vi "2024_day02.vi"() -> ()   [LabVIEW 2023]
uses:
  <userlib>/_OpenG.lib/string/string.llb/openg_string.lvlib
panel:
  out "Result - Task 2":i16
  out "Result - Task 1":i16
  in  "Switch":bool caption="Ex. Data  vs.  User Data"
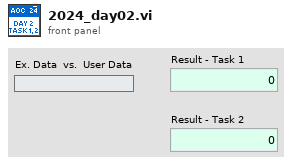
[diagram p1: front panel]
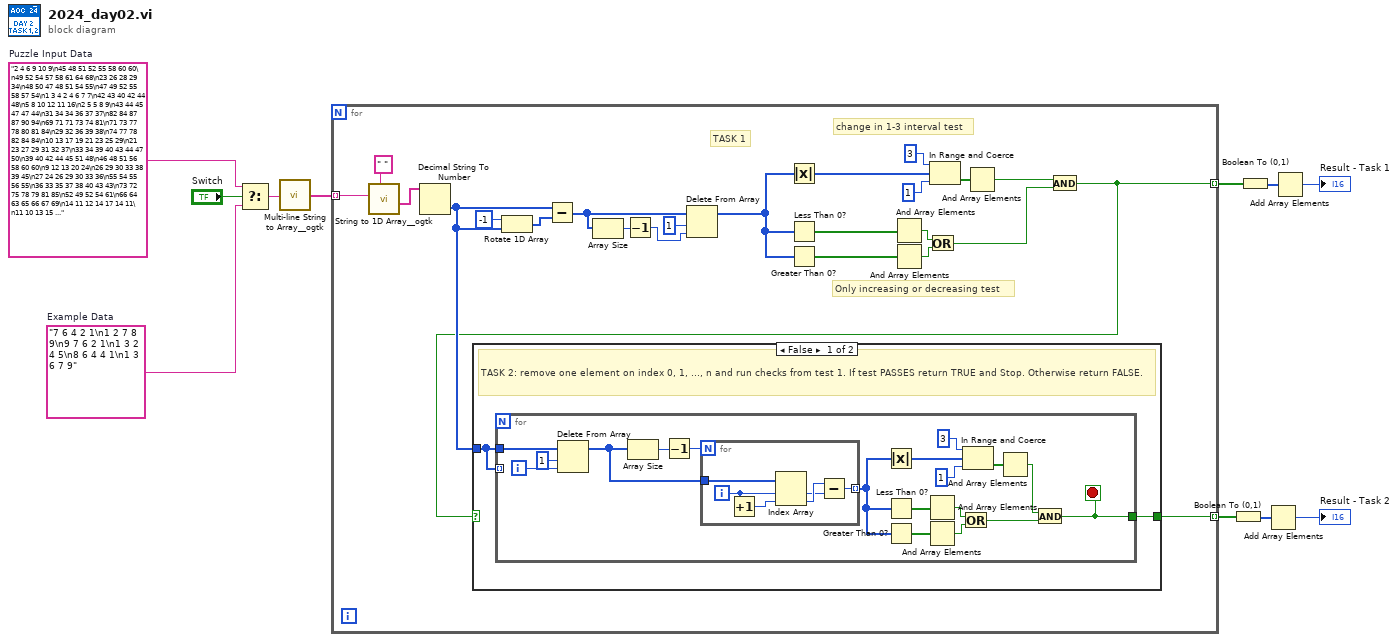
[diagram p0: block diagram]
diagram:
  w9 = "2 4 6 9 10 9\n45 48 51 52 55 58 60 60\n49 52 54 57 58 61 64 68\n23 26 28 29 34\n48 50 47 48 51 54 55\n47 49 52 55 58 57 54\n1 3 4 2 4 6 7 7\n42 43 40 42 44 48\n5 8 10 12 11 16\n2 5 5 8 9\n43 44 45 47 47 44\n31 34 34 36 37 37\n82 84 87 87 90 94\n69 71 71 73 74 81\n71 73 77 78 80 81 84\n29 32 36 39 38\n74 77 78 82 84 84\n10 13 17 19 21 23 25 29\n21 23 27 29 31 32 37\n33 34 39 40 43 44 47 50\n39 40 42 44 45 51 48\n46 48 51 56 58 60 60\n9 12 13 20 24\n26 29 30 33 38 39 45\n27 24 26 29 30 33 36\n55 54 55 56 55\n36 33 35 37 38 40 43 43\n73 72 75 78 79 81 85\n52 49 52 54 61\n66 64 63 65 66 67 69\n14 11 12 14 17 14 11\n11 10 13 15 14 14\n41 38 39 40 38 42\n91 88 86 87 92\n47 44 46 47 48 48 50\n91 89 92 93 93 90\n40 37 37 38 41 41\n60 59 60 63 65 68 68 72\n28 27 28 28 33\n74 71 73 74 76 80 81\n30 28 32 34 32\n51 50 53 54 55 58 62 62\n68 67 70 72 76 80\n17 14 15 19 25\n74 72 75 78 84 87 90 92\n34 32 38 41 42 41\n12 11 12 15 18 24 25 25\n75 74 75 78 79 86 90\n81 78 84 87 88 89 94\n72 72 73 76 78\n22 22 23 24 25 28 26\n47 47 49 50 53 55 55\n19 19 20 23 26 28 32\n23 23 26 27 28 30 32 39\n93 93 94 97 94 96 99\n80 80 83 84 87 84 81\n27 27 30 31 28 31 33 33\n18 18 21 18 22\n51 51 54 51 52 53 60\n24 24 24 27 30\n79 79 79 80 77\n81 81 84 84 86 89 89\n46 46 46 49 52 56\n46 46 46 47 48 54\n40 40 44 47 49 50 53 56\n42 42 45 49 52 54 51\n21 21 24 28 31 31\n66 66 70 71 74 78\n79 79 81 82 83 85 89 94\n18 18 21 26 27\n53 53 58 61 62 59\n57 57 59 61 67 67\n83 83 84 90 94\n4 4 6 11 17\n12 16 17 18 21 24 27 30\n28 32 35 36 38 37\n18 22 25 26 26\n74 78 81 84 86 89 93\n5 9 10 12 13 15 18 23\n57 61 60 63 66\n69 73 74 77 75 76 78 75\n30 34 31 32 32\n77 81 84 86 84 88\n8 12 14 13 15 18 20 26\n61 65 65 66 69\n3 7 10 10 13 15 12\n84 88 90 92 94 94 94\n19 23 26 29 30 30 34\n68 72 75 75 80\n58 62 66 69 71\n9 13 17 18 21 22 19\n7 11 15 16 19 22 22\n23 27 29 33 34 38\n62 66 68 72 78\n54 58 64 67 70 73 74 77\n69 73 78 81 78\n67 71 77 80 83 84 84\n70 74 75 80 84\n40 44 50 51 53 56 61\n65 70 73 75 77\n33 38 40 42 44 43\n43 50 52 53 53\n33 38 41 43 44 48\n72 79 82 85 87 89 92 99\n74 79 81 84 87 84 85\n13 19 21 18 19 16\n89 95 92 94 97 98 98\n35 41 44 47 48 46 50\n35 40 43 41 48\n8 14 16 18 18 19 20\n40 47 49 50 50 51 54 52\n21 26 28 29 29 30 33 33\n40 45 47 48 48 52\n48 53 55 55 61\n54 59 60 64 66 67 68\n35 42 44 46 47 51 49\n40 45 47 51 53 53\n17 22 26 27 31\n75 81 85 87 94\n44 50 57 60 63 65\n48 53 56 63 60\n47 52 54 59 61 61\n27 33 38 41 45\n66 71 72 77 80 83 90\n30 28 27 24 22 21 24\n17 16 15 13 11 8 7 7\n37 36 34 33 31 30 29 25\n93 91 90 87 80\n18 16 15 13 14 11\n77 74 71 70 67 69 70\n49 46 45 44 47 47\n80 79 77 76 77 74 70\n50 49 47 50 49 48 47 42\n86 83 80 80 77\n66 64 61 61 59 57 55 57\n62 60 58 58 55 53 53\n63 60 60 57 53\n59 57 57 56 53 50 48 41\n98 96 92 91 89 88 87\n98 95 91 89 86 88\n78 77 74 72 69 65 65\n15 13 12 10 9 5 1\n62 59 58 54 47\n99 98 97 92 89\n84 83 82 76 75 73 76\n47 44 39 36 35 33 33\n42 39 33 30 29 26 22\n34 32 31 29 27 21 19 13\n55 56 55 54 52\n86 89 88 85 82 83\n72 74 73 70 69 66 66\n70 72 70 68 65 63 60 56\n82 83 82 79 77 76 73 68\n38 41 44 43 40 38\n2 5 4 7 4 5\n79 81 80 83 83\n26 27 24 27 24 23 19\n22 25 26 23 21 18 16 9\n18 21 19 17 17 16\n52 55 53 53 50 49 51\n25 27 26 26 23 21 21\n9 11 8 8 4\n23 26 23 21 21 18 17 12\n54 55 53 51 47 45\n79 82 80 76 75 73 71 72\n69 71 67 64 62 60 60\n26 29 28 24 20\n71 74 70 69 67 64 58\n82 83 76 75 74 73 72\n79 82 80 75 73 75\n7 10 5 3 1 1\n84 87 86 80 78 75 71\n27 28 21 20 17 15 8\n90 90 89 86 84\n35 35 34 32 31 29 26 28\n57 57 55 54 52 49 49\n51 51 50 47 43\n65 65 63 61 59 58 57 52\n44 44 43 40 37 35 38 35\n24 24 22 20 18 21 18 19\n76 76 75 78 78\n39 39 36 39 36 35 31\n39 39 40 38 31\n28 28 25 22 22 19\n12 12 9 8 8 6 4 7\n19 19 16 16 16\n63 63 62 59 59 55\n87 87 87 85 78\n64 64 61 57 55 53 50\n61 61 58 54 56\n17 17 14 10 8 8\n48 48 46 42 41 40 39 35\n29 29 25 22 17\n60 60 57 55 52 47 44\n63 63 62 60 54 53 51 52\n98 98 92 91 91\n46 46 43 41 38 32 28\n37 37 32 29 26 23 21 14\n57 53 52 49 48 46 45\n85 81 79 78 76 78\n24 20 17 16 13 12 9 9\n39 35 34 32 28\n56 52 50 47 46 45 44 38\n13 9 11 9 6\n98 94 92 90 92 90 89 90\n28 24 25 22 20 20\n42 38 35 33 35 33 29\n23 19 17 18 17 14 12 6\n35 31 29 26 25 25 24 23\n23 19 16 14 11 8 8 11\n82 78 78 76 76\n44 40 40 37 33\n45 41 39 38 38 31\n77 73 70 68 64 63 62\n52 48 47 43 40 39 38 40\n74 70 66 63 63\n55 51 47 46 45 44 40\n71 67 64 63 59 58 57 52\n49 45 43 40 39 36 30 28\n44 40 37 35 29 31\n27 23 21 20 19 16 11 11\n55 51 46 45 41\n83 79 77 71 70 68 62\n16 9 7 4 3\n67 62 60 57 58\n30 24 21 19 18 17 14 14\n21 15 13 11 7\n27 22 20 19 16 13 11 5\n15 8 7 8 5\n53 46 43 40 41 38 39\n76 70 69 66 68 68\n39 32 34 32 29 26 25 21\n92 85 83 86 84 81 76\n27 20 18 17 16 16 15\n21 14 11 9 8 8 9\n27 22 21 21 19 19\n58 53 53 51 48 47 43\n66 59 56 56 53 46\n70 64 60 59 56\n48 43 40 39 35 38\n61 54 50 48 46 46\n72 67 63 62 61 60 56\n96 91 87 84 77\n60 55 50 48 47 45\n43 38 35 29 28 25 27\n94 89 88 86 84 78 77 77\n58 51 48 46 43 41 34 30\n35 29 26 20 13\n87 90 91 92 89\n9 10 11 13 15 15\n5 6 7 8 11 14 15 19\n61 64 66 68 69 76\n64 66 67 69 71 74 73 75\n13 14 17 16 18 17\n91 94 97 94 96 96\n87 88 87 88 90 93 97\n47 49 51 48 53\n29 30 33 35 38 40 40 41\n58 61 62 65 68 68 71 69\n4 6 9 9 9\n73 76 77 79 79 81 85\n30 32 34 34 39\n24 27 30 31 35 38 41\n69 72 76 78 77\n29 31 33 37 37\n66 68 70 72 76 80\n82 84 87 91 98\n68 71 74 79 81 84 86\n72 75 77 78 81 86 88 86\n11 14 20 21 21\n44 46 48 49 50 56 57 61\n31 34 35 38 40 41 48 53\n56 53 55 56 58 60\n56 53 56 59 61 62 61\n9 8 10 13 13\n7 4 5 8 9 11 15\n29 27 29 32 38\n10 8 10 11 10 13\n77 74 77 76 73\n80 79 81 83 82 84 84\n68 65 67 64 68\n45 44 41 44 46 47 50 57\n15 14 16 17 17 19 22 23\n28 26 27 27 25\n67 64 64 67 70 70\n10 7 10 12 12 13 17\n56 54 54 55 62\n23 20 22 26 27 30\n29 28 31 35 33\n21 19 23 25 25\n37 35 39 42 43 47\n60 57 61 64 69\n49 47 54 57 58 59 60\n76 74 79 81 78\n60 57 58 64 67 67\n59 57 64 65 69\n80 77 78 85 88 95\n72 72 73 75 77 78 81 84\n91 91 93 94 95 97 94\n62 62 65 68 71 74 74\n31 31 33 36 37 38 41 45\n80 80 83 85 87 88 91 96\n39 39 40 37 40 41 42\n87 87 85 88 90 88\n49 49 52 49 49\n50 50 51 52 50 54\n43 43 45 43 46 49 50 56\n43 43 43 46 48\n21 21 24 25 28 28 27\n3 3 3 4 7 8 11 11\n48 48 51 51 55\n62 62 65 67 70 72 72 79\n29 29 32 36 39 41\n37 37 41 43 44 46 44\n15 15 19 20 21 23 25 25\n71 71 75 78 82\n69 69 73 76 79 82 89\n84 84 86 87 94 96\n75 75 76 82 83 85 83\n44 44 45 48 51 57 57\n71 71 76 77 80 81 82 86\n84 84 90 91 96\n60 64 65 67 69 71\n46 50 52 53 55 58 57\n36 40 43 46 47 49 49\n28 32 35 38 39 43\n26 30 32 34 35 41\n21 25 28 25 28\n35 39 37 40 42 40\n37 41 43 40 42 42\n20 24 25 27 29 28 32\n46 50 53 54 52 54 59\n84 88 89 90 92 92 94\n55 59 59 60 62 65 62\n48 52 54 54 57 60 63 63\n63 67 69 70 72 72 75 79\n74 78 78 79 82 85 86 91\n64 68 71 75 77\n14 18 19 23 21\n47 51 55 58 61 61\n14 18 22 23 27\n72 76 77 78 81 85 86 91\n82 86 88 94 95 96 98\n39 43 46 53 56 54\n10 14 15 18 24 24\n70 74 75 78 85 87 91\n40 44 45 48 50 55 61\n4 11 12 14 16\n48 53 56 58 61 59\n32 37 40 41 41\n10 15 17 20 23 25 27 31\n78 84 86 87 89 90 97\n89 94 92 95 96\n41 46 49 51 52 53 50 47\n84 90 91 89 92 92\n61 66 64 66 68 70 74\n75 81 84 81 86\n13 18 18 21 24 26 29\n39 46 47 48 51 51 48\n12 19 19 21 21\n10 15 15 18 22\n72 78 80 82 82 87\n67 72 75 78 81 85 87\n56 63 67 70 73 72\n81 88 92 95 96 99 99\n1 7 8 12 13 15 19\n21 28 29 31 33 37 40 46\n44 51 52 59 60 63\n12 17 19 24 22\n35 41 46 49 52 54 56 56\n25 32 34 37 44 45 49\n47 52 55 62 67\n30 27 24 23 21 23\n72 69 68 66 65 63 61 61\n84 82 81 78 75 72 68\n86 83 81 79 78 75 70\n58 57 59 57 55\n14 13 11 13 12 9 11\n23 20 23 21 20 19 18 18\n66 64 62 63 59\n45 43 45 42 36\n42 39 37 37 35 33\n12 10 9 8 5 5 6\n56 53 53 51 51\n86 84 83 82 80 79 79 75\n87 84 81 78 78 72\n36 33 29 27 26 25\n73 72 71 69 65 62 64\n41 39 37 34 31 27 27\n51 50 49 46 45 41 37\n70 69 67 65 63 60 56 51\n81 78 76 73 72 70 64 61\n65 63 57 54 52 49 48 49\n53 50 48 42 40 39 39\n46 44 42 40 38 37 31 27\n65 64 63 57 55 53 52 45\n71 73 72 69 66 63 60 57\n62 65 64 63 60 57 56 57\n80 83 82 79 78 76 74 74\n73 74 71 69 68 67 63\n50 52 51 49 43\n14 16 14 11 8 11 8 7\n73 74 76 73 76\n7 10 7 8 5 4 1 1\n37 40 38 37 36 35 38 34\n72 75 72 74 72 71 68 62\n55 56 53 53 52\n2 4 4 2 5\n32 35 32 29 26 23 23 23\n79 81 81 80 77 76 73 69\n69 71 68 68 62\n23 24 22 18 16\n67 68 65 62 58 60\n17 20 16 13 11 11\n28 29 25 23 19\n87 90 86 83 81 76\n42 44 37 36 34 33\n9 10 8 3 2 1 2\n91 93 91 88 81 78 78\n33 36 34 28 27 23\n88 90 84 83 80 77 76 71\n26 26 25 22 19 16 14\n86 86 83 82 85\n65 65 63 60 59 57 55 55\n94 94 93 90 87 85 81\n31 31 30 29 27 22\n31 31 30 29 26 27 26 25\n77 77 76 75 72 73 76\n89 89 87 89 86 86\n80 80 81 80 76\n19 19 18 19 14\n99 99 96 95 95 93 90 89\n19 19 17 14 11 11 13\n18 18 18 15 13 13\n69 69 67 67 65 61\n90 90 87 87 85 83 76\n47 47 44 40 39\n12 12 10 6 4 2 4\n18 18 14 13 11 11\n67 67 63 60 56\n50 50 49 48 47 44 40 35\n51 51 44 41 38 36\n90 90 83 82 80 79 82\n56 56 54 53 48 47 46 46\n83 83 82 76 72\n24 24 21 15 10\n87 83 81 79 77 76 73\n93 89 88 87 84 86\n86 82 80 77 77\n26 22 19 18 14\n38 34 32 31 26\n48 44 45 44 41 39 36 34\n84 80 83 80 82\n99 95 97 95 94 94\n41 37 38 37 34 31 27\n56 52 49 51 50 47 40\n24 20 19 18 15 15 12\n74 70 68 67 66 66 65 67\n83 79 79 76 74 73 73\n49 45 42 41 39 36 36 32\n75 71 70 70 63\n18 14 10 9 6 3 2\n47 43 39 36 38\n54 50 47 45 42 38 37 37\n37 33 30 29 25 22 21 17\n78 74 70 68 65 62 57\n22 18 13 12 10 7 6\n35 31 28 27 26 19 18 21\n53 49 48 46 40 37 37\n81 77 76 69 68 65 61\n49 45 42 41 36 33 31 25\n47 40 37 35 34 32 29\n23 17 15 13 12 10 11\n90 85 83 82 81 81\n62 57 56 55 53 52 51 47\n68 61 60 58 57 54 47\n28 23 22 24 23 20 18\n96 91 90 88 87 85 86 87\n16 11 8 7 10 9 9\n98 93 92 95 94 90\n42 35 34 32 29 28 31 24\n44 39 37 34 34 33 31 30\n26 21 21 19 16 15 18\n90 84 82 80 78 76 76 76\n75 70 67 66 66 65 61\n31 24 24 23 16\n19 13 10 9 8 4 3\n73 66 65 61 59 56 55 58\n82 77 76 75 71 69 66 66\n71 65 61 59 55\n72 66 63 59 56 50\n75 68 65 63 57 55 54 51\n32 27 24 17 16 15 13 16\n41 34 27 26 23 23\n47 40 37 35 32 30 23 19\n68 62 57 55 52 51 49 43\n13 13 12 5 1\n39 36 38 42 43\n34 32 38 39 41 44 46 44\n95 98 96 94 92 89 86\n15 21 23 24 25 27 27\n13 11 12 15 14\n72 72 74 75 76 79 81 84\n93 87 83 82 83\n62 60 63 64 71 78\n26 26 28 30 33 37 35\n63 60 57 57 56 53 50 48\n33 38 41 43 47\n93 95 95 94 91 90 86\n60 65 67 64 65 66 69 69\n48 52 55 59 61 64 64\n9 14 15 17 17 20\n86 88 90 92 92 95 95\n61 55 53 53 56\n19 20 17 16 11\n46 52 54 59 57\n20 20 21 18 20 21 18\n73 74 77 75 76 79 77\n57 58 59 61 65 65\n97 97 95 92 89 82 82\n3 7 8 12 19\n54 57 58 62 65 68 71\n46 49 55 56 57 58 62\n82 78 77 78 74\n74 73 75 78 80 86\n85 85 83 82 82 82\n51 54 56 57 57\n17 16 14 11 11 8 6 9\n65 65 60 58 55 52 51 49\n3 7 8 15 18 20 18\n66 70 74 77 78 82\n67 67 67 64 62 64\n63 60 59 57 54 53 49\n44 51 53 56 58 57\n36 37 32 30 26\n50 53 50 45 42\n23 19 17 15 13 16 11\n81 77 71 69 69\n32 28 25 21 22\n68 71 74 77 81 86\n11 15 17 18 18\n86 86 85 84 79 77 75 78\n39 36 37 42 42\n10 10 7 5 3 1 1\n11 10 10 11 15\n85 78 77 77 75 69\n50 49 52 50 50\n19 14 11 10 8 7 4 4\n62 63 59 58 56 54 52 46\n74 70 70 69 65\n90 90 93 94 94 92\n50 49 48 45 43 42 42\n58 57 58 59 59 58\n24 19 18 16 15 8 6\n2 2 4 3 6 7 7\n61 63 60 61 61\n22 19 16 14 11 14 10\n10 16 19 23 24 27 34\n90 90 91 95 96\n32 36 38 38 40 40\n72 69 70 71 73\n60 64 62 65 71\n28 35 38 40 43\n26 19 17 15 11 8\n87 87 84 81 80 82\n76 80 84 86 85\n92 92 91 88 90 88 90\n56 63 65 66 68 70 72 77\n10 13 15 17 20 20 26\n14 16 14 11 7 6\n58 59 58 52 53\n33 31 30 23 21 18 12\n23 25 27 29 33\n59 63 65 63 64 65 69\n68 70 68 69 68 67\n98 98 95 92 87 84 79\n32 34 33 32 29 26 25 26\n70 64 62 61 60 59\n66 63 60 57 57 54 50\n86 84 82 80 77 73 71 67\n15 18 19 19 23\n29 25 22 19 17 14 11 5\n83 87 90 93 90 93 96\n64 62 60 57 59\n12 12 13 14 17 21\n61 68 69 68 74\n30 23 21 24 18\n70 66 66 64 62 59 59\n63 60 59 55 48\n96 96 98 95 95\n54 54 60 61 64 65 68 71\n54 55 58 59 65 67 69\n85 79 76 75 75 71\n93 87 86 84 77 76 74 77\n62 63 66 73 79\n78 81 84 86 87 86\n53 52 50 44 41 38\n13 17 19 22 24 28\n96 90 83 81 80 74\n69 69 71 77 77\n2 5 7 7 4\n45 45 43 40 34\n79 81 79 79 78 75 72\n86 84 87 88 90 92 95 95\n65 67 68 69 70 76\n53 50 52 56 57 58 60 67\n49 51 54 53 49\n42 39 41 44 47 44 46\n84 83 81 78 75 73 71 65\n89 83 82 85 84 82 79\n75 74 71 69 65 62\n29 30 32 33 38 36\n33 26 23 22 15 11\n39 32 30 28 27 26 20\n48 48 50 51 52 56 56\n58 52 49 46 45 41 34\n94 93 91 89 89 87 85 80\n84 87 90 90 92 93\n21 21 19 21 15\n37 37 35 33 29\n65 62 61 64 65 66 63\n58 58 61 62 67 69 70 68\n26 26 31 33 37\n59 65 66 68 75 79\n6 12 13 15 19 22 24 28\n38 38 39 42 43 42 45 49\n44 44 40 39 35\n81 77 76 73 76 73 70\n25 28 27 23 24\n20 20 23 20 16\n18 22 25 24 26 26\n59 61 60 63 64 68\n72 76 79 81 84 86 90 92\n46 46 49 49 51 52 56\n89 85 83 82 82 83\n5 12 14 18 18\n63 63 62 61 60 60 57 51\n53 49 48 46 44 41 37\n26 22 19 17 14 12 10 12\n78 82 83 85 87 90 90 91\n43 42 37 36 34 31 31\n85 82 80 79 81 80\n84 87 89 86 80\n35 29 28 25 23 19 19\n30 26 24 23 23 21 19\n37 37 34 32 32 29 27 23\n95 97 99 96 96\n40 36 34 33 29 28 24\n21 21 22 25 28 35\n91 91 89 88 84 82 79 80\n80 85 88 90 92 90 87\n81 79 80 81 80 81 83 87\n31 31 32 31 29 27\n21 14 13 14 12 8\n66 66 64 61 59 59 57 56\n33 35 32 30 29 29 32\n94 91 89 91 97\n29 35 40 41 44 50\n73 77 78 84 85 88 94\n25 27 24 24 19\n37 41 43 40 41 44 47 45\n29 23 20 19 15 14 12 8\n87 87 90 93 93\n78 80 81 80 83\n25 27 26 25 22 18\n84 80 79 74 71 67\n37 39 43 46 49 50 49\n68 67 70 70 72 73 76 83\n95 95 93 89 88\n13 18 15 18 21 24 27 31\n8 12 15 16 16 17 22\n38 37 40 42 42 45 46\n28 28 28 30 31 33\n93 94 92 93 95 96 97\n14 12 12 15 16 16\n19 23 24 29 32\n81 81 82 84 87 88 92 98\n95 91 86 84 83 80\n25 23 23 20 18 18\n21 20 17 13 16\n57 59 56 53 51 44 44\n95 89 87 84 83 81 75 75\n22 22 23 25 25 26 26\n5 5 7 9 10 14 16 20\n58 54 52 51 50 48 48\n26 22 19 18 12 9 8 9\n48 44 42 41 34 29\n56 56 58 56 59 61 62 63\n12 16 18 20 22 22 21\n55 58 61 65 67 68 69 73\n43 43 40 38 35\n34 28 25 22 24 21 19 19\n7 13 14 17 20 21 25 28\n54 59 61 64 67 70 70 77\n28 24 21 21 15\n73 70 69 68 71 69 72\n71 64 62 64 61 64\n49 50 49 48 44 43 41 37\n55 59 61 63 66 68\n77 73 72 68 67 66 66\n82 83 86 84 85 86 88 95\n28 28 27 24 20 17 12\n50 54 54 56 60\n21 22 19 17 17 15 12 12\n74 70 69 68 71 69 69\n12 16 23 24 28\n77 74 71 69 64 67\n18 22 23 30 33 33\n11 12 17 18 18\n11 8 11 12 13 14 18 18\n51 58 57 58 61\n74 68 65 63 66\n11 11 13 15 16 19 22 21\n83 80 79 78 75 73 71 68\n76 74 73 70 67\n96 94 91 90 88\n18 20 22 23 25\n60 63 64 67 69 71 74\n15 16 18 21 24 27\n20 18 15 13 10\n64 62 59 57 56 53 50\n34 37 40 43 45\n4 7 9 12 14\n18 19 20 22 25 27 29 32\n67 64 63 60 59 57 56 55\n25 23 21 18 17 16 14\n15 18 20 22 25 28 30\n94 91 89 88 85 84\n83 85 86 87 89\n82 85 86 87 90 91 93 95\n73 70 67 65 62 59 56 53\n78 81 84 85 88\n94 92 89 88 87\n90 87 85 83 81 80 79 76\n29 30 33 36 38 39 41 44\n37 40 41 42 45 46 48 49\n29 30 31 33 34 35\n29 26 23 21 18 15\n14 12 11 10 9 6 5\n65 63 60 57 54\n40 39 38 37 35 33 32 31\n49 51 53 54 55\n43 46 48 49 50\n3 6 8 10 12\n25 22 21 19 18 15 13\n23 25 27 29 31 34 35 38\n45 46 47 49 50\n55 58 60 62 65 68 69 70\n53 55 58 61 63 64 65\n69 66 64 63 62\n80 83 84 85 86 88 91\n52 54 55 57 59 61 63 66\n27 30 33 36 37 38 40\n90 89 87 86 84 82\n32 34 36 37 39 40 41 42\n89 86 83 81 80 79 78\n21 20 19 17 14\n77 78 79 80 82 83 84\n81 82 85 86 88 90 93 96\n68 70 71 74 76 77 79\n41 39 38 37 35 32 31\n40 43 45 47 48 49 51\n89 88 86 85 84 82 79\n14 15 17 18 21 22 25 27\n79 77 74 73 72 71 69 68\n73 76 78 81 84 87 90 92\n78 81 84 87 90 93\n33 31 29 27 25 22 21\n65 64 62 59 57 54\n81 83 86 87 90\n27 30 33 35 38 39 42 45\n59 56 53 50 49 47\n68 65 63 62 61 58 56 54\n55 52 49 47 45 43 40\n83 85 87 90 91\n76 73 72 71 68 65 64 63\n43 44 46 49 52\n18 21 23 26 27 28 31 33\n84 81 79 77 76 74\n13 15 17 20 22 24 27 30\n12 15 18 21 22\n60 59 56 53 51 48 47 45\n59 60 62 63 66 69 70\n48 46 43 42 41 38 37\n54 51 48 45 42 39 36 34\n61 62 63 64 66 67\n22 23 26 28 30\n37 36 33 30 27 26\n68 65 62 59 56\n19 22 24 26 27 28 30 33\n36 37 39 42 44 45 47\n65 62 59 56 53\n42 45 47 48 50\n58 57 55 52 51\n34 36 38 40 43 44 45\n5 6 8 10 11 14\n88 86 84 81 79 77\n27 26 23 22 20 17 16\n73 71 70 68 65 63 62\n62 64 67 70 71 73 76 79\n57 60 61 63 64\n99 98 96 95 94\n37 35 34 33 32 30 29 27\n87 84 82 80 77\n61 63 65 66 68 71 73 74\n25 22 20 18 16 13 11 8\n22 19 18 15 12 10 7 5\n97 96 95 94 93 92 91 88\n82 83 86 87 90 91 92 94\n46 48 49 50 51\n53 51 50 47 44 42\n41 42 45 46 48 49 51\n87 85 84 83 82 81\n24 21 18 17 14 11 10\n27 25 24 22 20 17\n14 12 11 9 7 6 5\n21 24 26 27 28 31 33\n13 12 9 8 7\n33 34 35 38 40 43\n84 81 78 77 74 71 68\n15 16 18 20 21 23 24\n24 21 18 17 14 12\n87 84 82 80 79 77\n94 91 90 88 85 82 79\n53 52 51 49 47 44 42\n43 42 40 39 38 37 34 31\n25 27 29 32 33 35 38\n40 37 34 33 31 29 28\n88 89 91 92 95 98\n74 75 77 80 83 84 85 86\n16 19 21 22 24\n59 58 55 53 52\n48 51 52 53 55 58 59\n27 28 31 32 33 36\n54 56 57 60 62 65 66\n25 26 29 30 33 36 37 39\n35 32 30 27 26 23 20 18\n36 37 40 43 44 45 46\n47 44 41 38 36 35\n64 62 60 58 55 52\n56 57 60 62 63 65 68\n20 21 22 23 26\n95 94 91 90 88 86 85\n95 94 91 88 86 85\n61 58 56 53 50 47\n83 85 86 88 91\n29 26 25 22 19 18 16 15\n76 74 72 69 66 63\n25 26 28 30 32\n66 65 63 61 58 57\n12 14 15 18 21 22\n52 51 48 47 46 43 40\n13 15 16 17 18 19\n60 63 64 65 67 68 69\n15 13 10 8 6 4 2\n53 54 57 59 61 62 65\n75 78 79 81 84 85\n27 26 25 22 19\n13 15 16 18 19 20 22\n96 93 90 87 84 81 79\n73 72 69 66 64 63 60 57\n20 22 25 28 29 32 33 35\n34 33 32 29 26\n89 88 87 84 82 80 78\n8 10 12 14 15 18 21 23\n34 35 36 37 39 41 44\n44 46 47 50 53 55 56 59\n49 46 44 42 41\n15 18 20 23 25 27\n39 41 43 44 47 48 50 53\n93 92 91 89 86 84 83 80\n34 32 29 28 26 23 21 18\n61 60 58 55 53 50\n46 44 42 39 37 36 33\n23 21 19 17 16 15 12 9\n5 7 8 9 10 12 15 16\n98 96 94 93 91 90 87 85\n92 91 88 87 86 83 82\n83 84 86 89 90 93 95 96\n87 89 90 91 93\n11 14 17 18 21 23 25\n7 8 9 12 14\n28 29 32 34 37 40 43 46\n81 83 84 86 87\n1 3 5 7 8\n59 58 56 55 54\n66 65 62 61 59 58\n92 89 87 84 82 79\n4 6 7 10 12 13 14\n43 46 47 50 53 55\n55 56 59 60 61 62\n65 64 63 61 60 59 58\n14 16 18 20 22 24\n89 91 93 96 98\n56 59 60 63 66 68 69 72\n32 35 36 37 39 40 42\n79 78 77 75 72\n60 62 65 66 68 71 73 76\n90 87 84 83 82 80 78 75\n38 40 43 44 47 49 52\n56 55 53 51 50 48 46\n70 68 66 64 61 59 57\n32 35 37 38 41 44 45 48\n21 24 26 29 32 34 36 38\n25 23 21 19 17 14\n36 35 34 32 31 29 26\n73 74 77 80 82 84 87 88\n22 20 17 16 13 12 11\n50 51 53 54 56 59 61\n8 11 14 16 18\n94 93 91 88 86 84\n84 87 88 90 92 95\n78 77 74 72 70 69\n46 44 43 40 37 36 33\n22 23 25 28 31 34\n72 70 68 65 64\n22 24 27 30 33\n70 69 67 65 62 60\n53 52 49 48 47\n28 26 23 22 19 16\n24 22 21 19 16 14 12 11\n44 41 40 37 35\n33 35 37 40 41 44 45 46\n40 37 35 33 32\n74 75 78 81 82 85\n72 74 76 79 80 81 82\n78 81 84 87 90 93 95 98\n44 45 48 51 52 54 56\n78 76 74 72 71 68 66 65\n86 85 84 82 81\n62 65 66 67 69\n11 13 16 19 20 22 25\n3 4 7 10 13 14 15\n18 16 13 10 8 5 4 2\n81 78 75 74 71 70 68 66\n49 46 44 43 42 41\n57 60 63 64 67 69 70\n18 15 12 11 9 8 5\n17 14 13 11 9 6\n21 24 27 30 32 35\n34 36 37 38 41 43 46\n83 82 79 78 75 73 71\n27 30 33 34 35 38 39 40\n74 75 77 78 79\n77 79 81 82 84 85 86\n77 74 72 69 68 67 65\n80 78 77 75 74\n16 19 22 25 27 29 32 34\n80 78 76 74 73\n35 33 31 30 28 26 24\n41 44 46 49 50 52 53\n52 54 56 57 60 61 62 63\n34 35 36 39 41 42 43 46\n73 76 77 79 82\n82 84 87 89 90 92\n67 65 62 60 57 56 55 52\n39 36 35 34 33 31 29\n40 39 36 33 32\n69 70 71 73 76 77 79\n46 49 52 54 57\n63 60 59 57 55 52\n47 44 42 40 38 37 34\n33 30 27 26 23 22\n16 18 20 22 23 26 29 30\n3 4 6 8 11 13 14 17\n8 11 14 16 18 20 22\n13 11 9 6 4\n35 33 30 28 27\n6 7 9 12 14 17 18 19\n77 74 71 69 67 66 64 61\n59 58 55 52 50 49\n69 71 74 76 79 82 85 87\n80 79 76 75 74\n75 72 70 67 64 63 61\n60 58 57 56 53 51 50 47\n21 24 26 28 30 31\n21 22 24 25 27 28 31\n98 96 94 93 90 87\n48 51 54 55 57\n83 86 88 89 91 93 94 97\n71 68 66 64 63 60 59\n34 36 37 40 43 45\n11 14 16 17 18 21 23 24\n97 94 91 88 85 83\n59 56 55 54 53 50 47\n68 65 62 60 57 55\n46 44 41 38 36 35\n42 39 37 34 31 29 27\n41 43 45 46 47 50 52 54\n85 84 82 81 80\n96 95 94 93 91 88 86 85\n71 73 75 77 80 81 84\n5 6 7 10 11 12 13 14\n14 11 8 5 4 3\n29 31 34 35 38 41 44 47\n68 70 72 73 76 78 80\n51 54 57 58 61 64\n93 91 90 89 86 83 80 77\n44 45 46 48 50 52\n71 73 75 76 79 81 84 86"  # Puzzle Input Data
  w10 = "7 6 4 2 1\n1 2 7 8 9\n9 7 6 2 1\n1 3 2 4 5\n8 6 4 4 1\n1 3 6 7 9"  # Example Data
  n1 = Select(t=w9, s="Switch", f=w10) -> (s? t:f=w5:string)
  n2 = call <userlib>:"Multi-line String to Array__ogtk.vi"("string"=w5) -> ("lines"=w8:string[])
  n3 = for {
    tunnel: w8 -> [w34] mode=indexing
    tunnel: [w13] -> w4 mode=indexing
    tunnel: [w12] -> w2 mode=indexing
    # "TASK 1"
    # "Only increasing or decreasing test"
    # "change in 1-3 interval test"
    n4 = call <userlib>:"String to 1D Array__ogtk.vi"("delimiter (Tab)"=" ", "string"=w34) -> ("Array of Strings"=w32:string[])  [unwired: 9 in]
    n5 = Decimal String To Number(string=w32) -> (number=w14:i32[])  [unwired: 2 in, 1 out]
    n6 = Rotate 1D Array(1:w14, 2:-1 ("n")) -> (0:w31:i32[])
    n7 = Subtract(x=w14, y=w31) -> (x-y=w29:i32[])
    n8 = Array Size(array=w29) -> (size(s)=w28:i32)
    n9 = Decrement(x=w28) -> (x-1=w22:i32)
    n10 = Delete From Array(array=w29, length=1 ("new element/subarray"), index=w22) -> (array with subset deleted=w19:i32[])  [unwired: 1 out]
    n11 = Absolute Value(x=w19) -> (abs(x)=w25:i32[])
    n12 = Less Than 0?(x=w19) -> (x < 0?=w16:bool[])
    n13 = Greater Than 0?(x=w19) -> (x > 0?=w15:bool[])
    n14 = And Array Elements(Boolean array=w16) -> (logical AND=w17:bool)
    n15 = And Array Elements(Boolean array=w15) -> (logical AND=w24:bool)
    n16 = Or(x=w17, y=w24) -> (x .or. y?=w20:bool)
    n17 = In Range and Coerce(upper limit=3 ("new element/subarray"), x=w25, lower limit=1 ("new element/subarray")) -> (In Range?=w18:bool[])  [unwired: 1 out]
    n18 = And Array Elements(Boolean array=w18) -> (logical AND=w21:bool)
    n19 = And(x=w21, y=w20) -> (x .and. y?=w13:bool)
    n20 = case shown="False" w13 {
      selector: w13 -> [_ w61]
      tunnel: w14 -> [w35 _]
      tunnel: [w36 w61] -> w12
      frame False {
        # "TASK 2: remove one element on index 0, 1, ..., n and run checks from test 1. If test PASSES return TRUE and Stop. Otherwise return FALSE."
        n21 = for {
          tunnel: w35 -> [w52]
          tunnel: [w37] -> w36
          tunnel: w35 -> [_] mode=indexing
          i -> [w49]
          stop <- w37 stop-if-true
          n22 = Delete From Array(array=w52, length=1, index=w49) -> (array with subset deleted=w51:i32[])  [unwired: 1 out]
          n23 = Array Size(array=w51) -> (size(s)=w54:i32)
          n24 = Decrement(x=w54) -> (x-1=w53:i32)
          n25 = for {
            N: w53 -> [_]
            tunnel: w51 -> [w60]
            tunnel: [w55] -> w39 mode=indexing
            i -> [w58]
            n26 = Increment(x=w58) -> (x+1=w59:i32)
            n27 = Index Array(array=w60, index #1=w58, index #2=w59) -> (element #1=w56:i32, element #2=w57:i32)
            n28 = Subtract(x=w57, y=w56) -> (x-y=w55:i32)
          }
          n29 = Absolute Value(x=w39) -> (abs(x)=w42:i32[])
          n30 = Less Than 0?(x=w39) -> (x < 0?=w47:bool[])
          n31 = Greater Than 0?(x=w39) -> (x > 0?=w48:bool[])
          n32 = And Array Elements(Boolean array=w47) -> (logical AND=w46:bool)
          n33 = And Array Elements(Boolean array=w48) -> (logical AND=w43:bool)
          n34 = Or(x=w46, y=w43) -> (x .or. y?=w44:bool)
          n35 = In Range and Coerce(upper limit=3 ("new element/subarray"), x=w42, lower limit=1 ("new element/subarray")) -> (In Range?=w45:bool[])  [unwired: 1 out]
          n36 = And Array Elements(Boolean array=w45) -> (logical AND=w38:bool)
          n37 = And(x=w38, y=w44) -> (x .and. y?=w37:bool)
        }
      }
      frame True {
        # "TASK 2: TURE -> pass thru only (no correction needed)"
      }
    }
  }
  n38 = Boolean To (0,1)(Boolean=w2) -> (0, 1=w3:i16[])
  n39 = Boolean To (0,1)(Boolean=w4) -> (0, 1=w7:i16[])
  n40 = Add Array Elements(numeric array=w3) -> (sum=→"Result - Task 2":i16)
  n41 = Add Array Elements(numeric array=w7) -> (sum=→"Result - Task 1":i16)
